vi "Module Name List FGV.vi"(7 "Action":T1, 9 "Module ID in":i32, 10 "Name":string) -> (1 "Module ID out":i32)   [LabVIEW 2017, in "SSH.lvlib"]
uses:
  SSH.lvlib
  Module Names FGV Actions.ctl
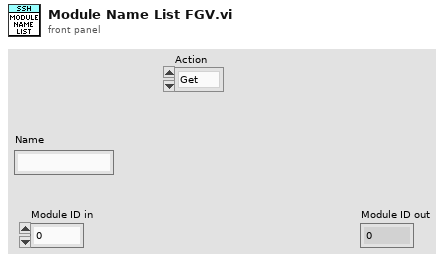
[diagram p1: front panel]
types:
  T1 = typedef "Module Names FGV Actions.ctl" = enum16{"Get", "Set"}
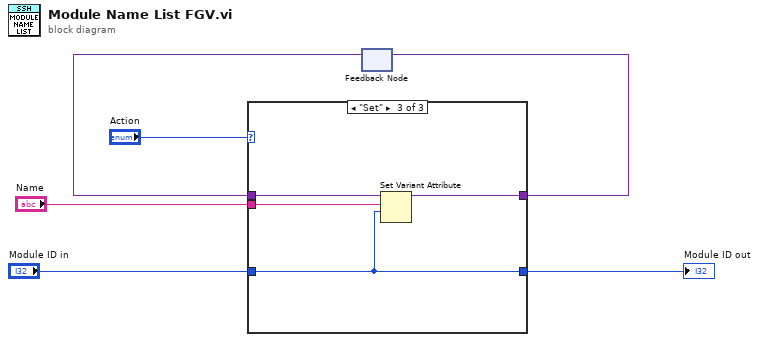
[diagram p0: block diagram]
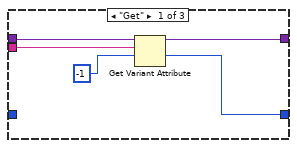
[diagram p2: hidden frame]
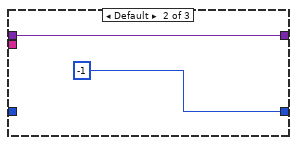
[diagram p3: hidden frame]
diagram:
  n1 = feedback #1() -> (w4:variant)  [unwired: 1 in]
  n2 = case shown="\"Set\"" "Action" {
    tunnel: [w10 w13 w17] -> w5
    tunnel: w4 -> [w11 w13 w16]
    tunnel: "Name" -> [w9 _ w15]
    tunnel: "Module ID in" -> [_ _ w14]
    tunnel: [w7 -1 ("Module ID in") w14] -> w1
    frame "Get" {
      n3 = Get Variant Attribute(Variant=w11, name=w9, default value (empty Variant)=-1 ("Module ID in")) -> (duplicate Variant=w10:variant, value=w7:i32)  [unwired: 1 in, 2 out]
    }
    frame Default {
    }
    frame "Set" {
      n4 = Set Variant Attribute(Variant=w16, name=w15, value=w14) -> (Variant out=w17:variant)  [unwired: 1 in, 2 out]
    }
  }
  "Module ID out" <- w1
  n5 = feedback-in #1(w5) -> ()
